vi "StitchTestLO.vi"() -> ()   [LabVIEW 2014]
uses:
  <vilib>/picture/picture.llb/Draw True-Color Pixmap.vi
panel:
  in  "SaveBmp":bool
  out "Intensity Graph":u32[][](graph)
  out "Yind":i32[](array[numeric])
  out "Xind":i32[](array[numeric])
  out "filenames":string[](array[string])
  in  "PathToVK4":path
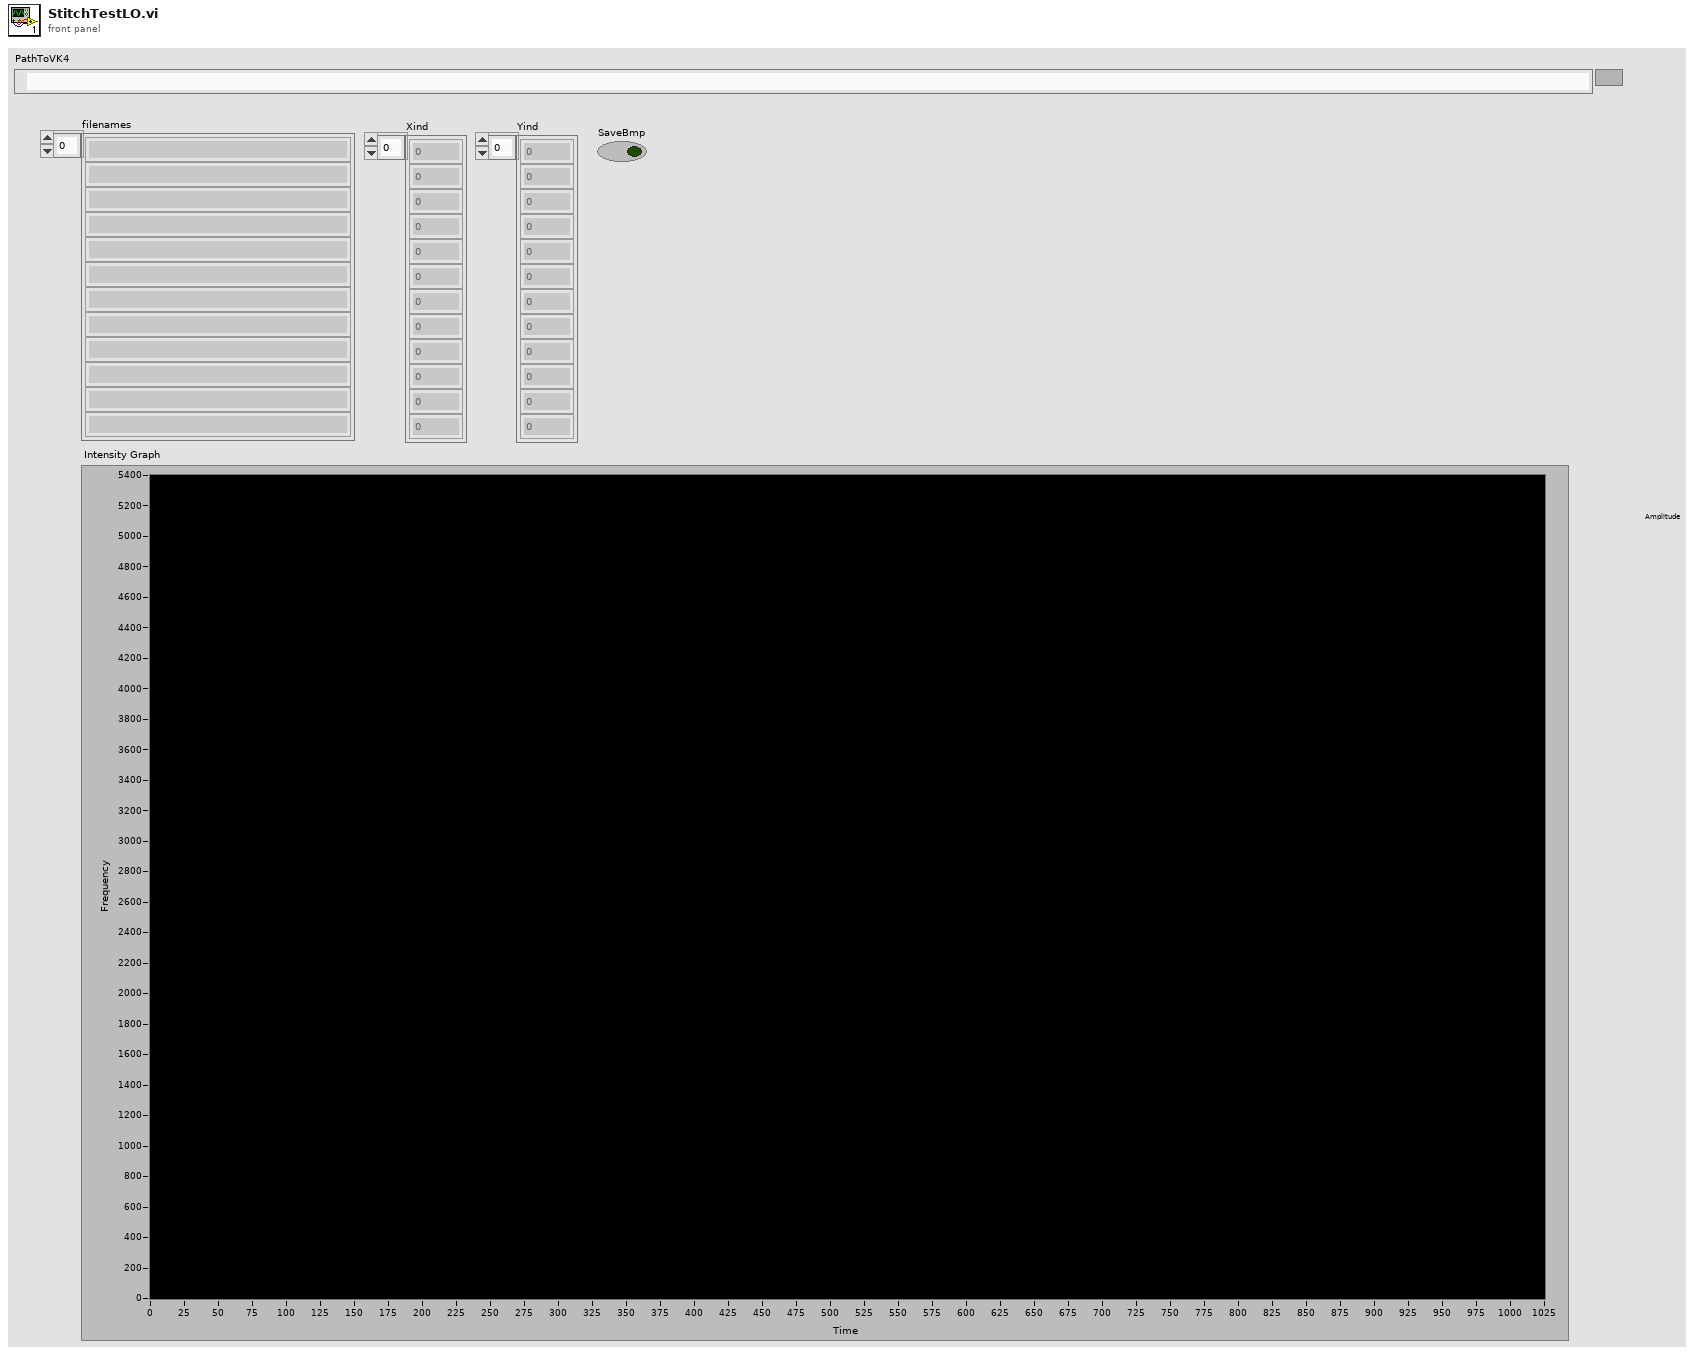
[diagram p1: front panel]
types:
  T1 = cluster{"left":i16, "top":i16, "right":i16, "bottom":i16}
  T2 = typedef "imagedata.ctl" = cluster{"image type":i32, "image depth":i32, "image":u8[], "mask":u8[], "colors":u32[], "Rectangle":cluster{"left":i16, "top":i16, "right":i16, "bottom":i16}}
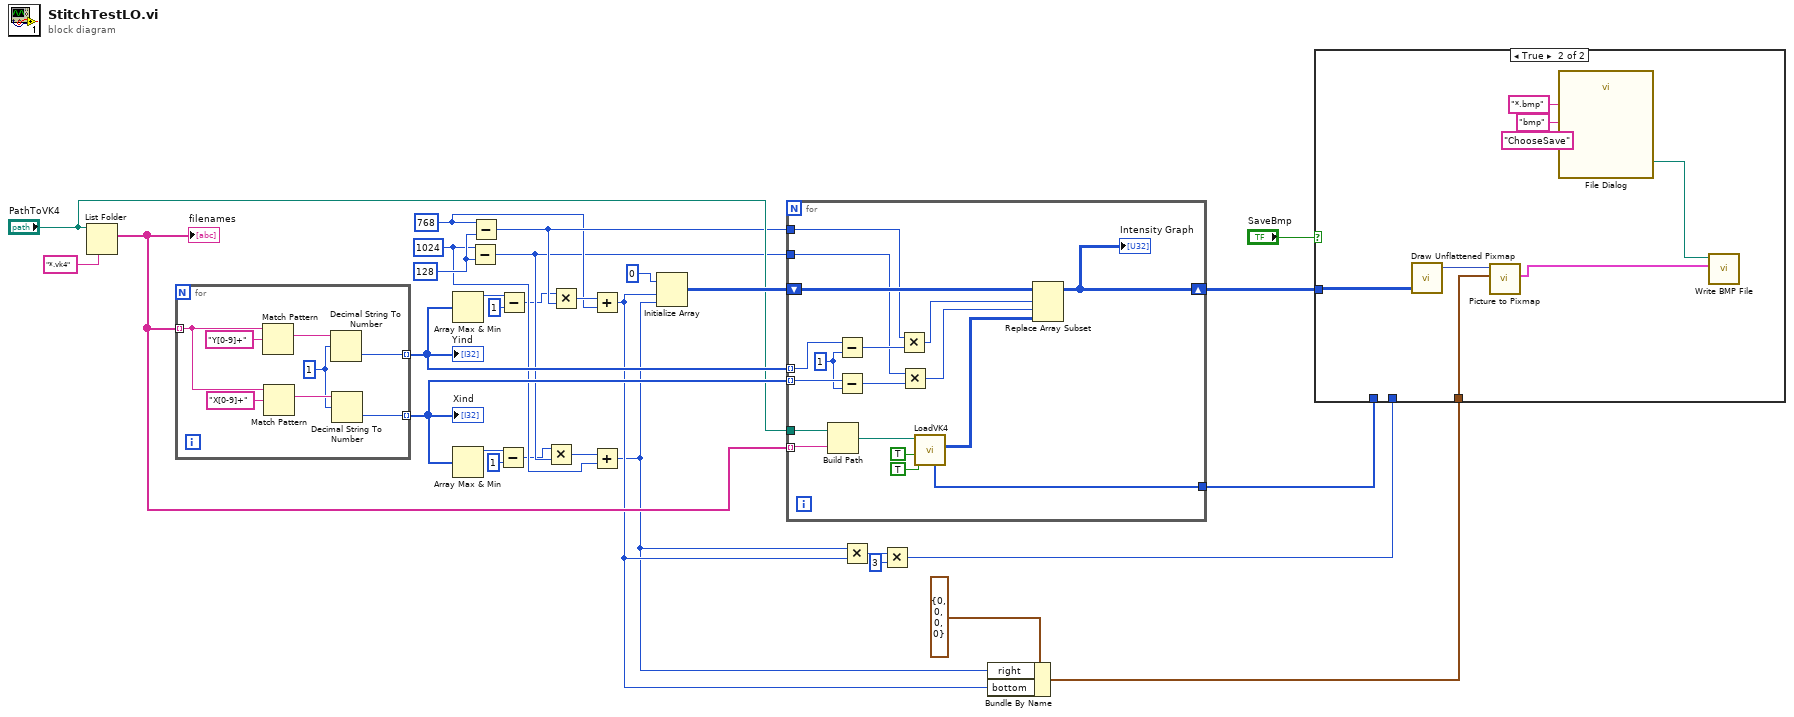
[diagram p0: block diagram]
diagram:
  w19 = 768
  w22 = 128 ("y")
  w18 = 1024
  n1 = List Folder(path="PathToVK4", pattern="*.vk4") -> (filenames=w27:string[])  [unwired: 2 in, 3 out]
  "filenames" <- w27
  n2 = for {
    tunnel: w27 -> [w34] mode=indexing
    tunnel: [w32] -> w25 mode=indexing
    tunnel: [w31] -> w24 mode=indexing
    w33 = 1 ("offset")
    n3 = Match Pattern(string=w34, regular expression="Y[0-9]+") -> (match substring=w37:string)  [unwired: 1 in, 3 out]
    n4 = Match Pattern(string=w34, regular expression="X[0-9]+") -> (match substring=w36:string)  [unwired: 1 in, 3 out]
    n5 = Decimal String To Number(string=w37, offset=w33) -> (number=w32:i32)  [unwired: 1 in, 1 out]
    n6 = Decimal String To Number(string=w36, offset=w33) -> (number=w31:i32)  [unwired: 1 in, 1 out]
  }
  "Xind" <- w24
  "Yind" <- w25
  n7 = Array Max & Min(array=w25) -> (max value=w9:i32)  [unwired: 3 out]
  n8 = Array Max & Min(array=w24) -> (max value=w5:i32)  [unwired: 3 out]
  n9 = Subtract(x=w18, y=w22) -> (x-y=w17:i32)
  n10 = Subtract(x=w19, y=w22) -> (x-y=w20:i32)
  n11 = Subtract(x=w5, y=1) -> (x-y=w4:i32)
  n12 = Subtract(x=w9, y=1) -> (x-y=w8:i32)
  n13 = Multiply(x=w4, y=w17) -> (x*y=w29:i32)
  n14 = Multiply(x=w8, y=w20) -> (x*y=w30:i32)
  n15 = Add(x=w30, y=w19) -> (x+y=w11:i32)
  n16 = Add(x=w29, y=w18) -> (x+y=w10:i32)
  n17 = Initialize Array(u32 0, w11, w10) -> (w26:u32[][])
  n18 = for {
    tunnel: w27 -> [w56] mode=indexing
    tunnel: "PathToVK4" -> [w55]
    tunnel: w25 -> [w51] mode=indexing
    tunnel: w24 -> [w50] mode=indexing
    tunnel: w17 -> [w44]
    shift-right: [w42] -> w16
    shift-left: w26 -> [w46]
    tunnel: w20 -> [w45]
    tunnel: [w43] -> w15
    w49 = 1 ("y")
    n19 = Build Path(base path=w55, name or relative path=w56) -> (appended path=w54:path)
    n20 = Subtract(x=w51, y=w49) -> (x-y=w48:i32)
    n21 = Subtract(x=w50, y=w49) -> (x-y=w47:i32)
    n22 = Multiply(x=w45, y=w48) -> (x*y=w41:i32)
    n23 = Multiply(x=w44, y=w47) -> (x*y=w40:i32)
    n24 = call "LoadVK4.vi"("SaveRaw"=TRUE, "SavePics"=TRUE, "PathToVK4"=w54) -> ("RGBarray2"=w39:u32[][], "IntenLU"=w43:u32[])  [unwired: 4 in, 3 out]
    n25 = Replace Array Subset(array=w46, new element=w39, index (row)=w41, index (col)=w40) -> (w42:u32[][])
    "Intensity Graph" <- w42
  }
  n26 = Multiply(x=w10, y=w11) -> (x*y=w3:i32)
  n27 = Multiply(x=w3, y=3) -> (x*y=w1:i32)
  n28 = Bundle By Name(cluster=T1 {"left"=0, "top"=0, "right"=0, "bottom"=0} ("Rectangle"), "right"=w10, "bottom"=w11) -> (w12:T1)
  n29 = case shown="True" "SaveBmp" {
    tunnel: w16 -> [_ w60]
    tunnel: w15 -> [_ _]
    tunnel: w1 -> [_ _]
    tunnel: w12 -> [_ w58]
    frame False {
    }
    frame True {
      n30 = call-poly <vilib>:"Draw Unflattened Pixmap.vi"("data (RGB format)"=w60) -> ("new picture"=w59:picture)  [unwired: 8 in]
      n31 = call <vilib>:"Picture to Pixmap.vi"("rect"=w58, "picture"=w59) -> ("image data"=w57:T2)  [unwired: 8 in, 1 out]
      n32 = call "File Dialog"("prompt"="ChooseSave", "pattern (all files)"="*.bmp", "pattern label"="bmp") -> ("selected path"=w61:path)  [unwired: 9 in, 3 out]
      n33 = call <vilib>:"Write BMP File.vi"("image data"=w57, "path to BMP file"=w61) -> ()  [unwired: 8 in, 2 out]
    }
  }
